vi "SwissSPAD Live_Decode SS2 FPGA Data_DVI.vi"(7 "SwissSPAD Live Gate Image Data Q":refnum<queue>, 8 "Error In":errorcluster, 9 "Buffer Size (#8-bit Images)":i32, 10 "SwissSPAD Live Internal Variables":T1={"okCFrontPanelDevices Refnum"=refnum, "Bottom Device Refnum"=refnum, "Display Image"=refnum, "# Live Images"=0, "relative s"=0.0, "# Image Sets"=0, "Message"="", "Current Image Set"=0, "# Datasets in Series"=0, "Current Dataset"=0, "Live Mode"=FALSE, "Recording Mode"=FALSE, "Record Button"=refnum, "\nLive Button"=refnum, "SwissSPAD Live Gate Image Data Q Name"="SS2 Live Gate Data Q", "Discard First Image"=FALSE, "Image Information"={"Save ROI Only"=FALSE, "Left"=0, "Top"=0, "Right"=0, "Bottom"=0, "Use Current ROI"=FALSE}, "Image Binning Options"={"Use Image Binning"=FALSE, "X Bin"=1, "Y Bin"=1}, "Bottom FPGA Serial Number"="", "Detector PCB Version"=enum."SS2 PCB1", "# Acquisitions"=1, "10 bits"=FALSE, "Top FPGA Serial Number"="", "Top Device Refnum"=refnum, "okCFrontPanel Refnum"=refnum} {"# Acquisitions" min=1; "Image Binning Options"."Y Bin" min=1; "Image Binning Options"."X Bin" min=1}, 11 "FPGA Data Q":refnum<queue>) -> ()   [LabVIEW 2021]
uses:
  SwissSPAD Live_Internal Variables.ctl
  D:/UCLA Thinkpad Google Drive/LabVIEW 2021 SP1/builds/SwissSPAD Live Distribution/Opal Kelly/C# Wrapper/v5.0.2/libFrontPanel-csharp.dll
  Opal Kelly/C# Wrapper/v5.0.2/libFrontPanel-csharp.dll
  <vilib>/vision/Image Controls.llb/IMAQ Image.ctl
  SwissSPAD Live_Image ROI Information.ctl
  Phasor/Image Binning Options.ctl
  SwissSPAD Live_SSx PCB Version.ctl
  8d2e2152-5180-46c7-ad9e-0233ef769053.vi
  LV Tools/Logical Processors Used.vi
  <vilib>/vision/NI_Vision_Development_Module.lvlib
  Notebook/Notebook.lvlib
  Rich Text Box/Rich Text Box.lvlib
panel:
  out "Activate Trigger Error Out":errorcluster
  out "8-bit Image Count":i32
  out "Error Out":errorcluster
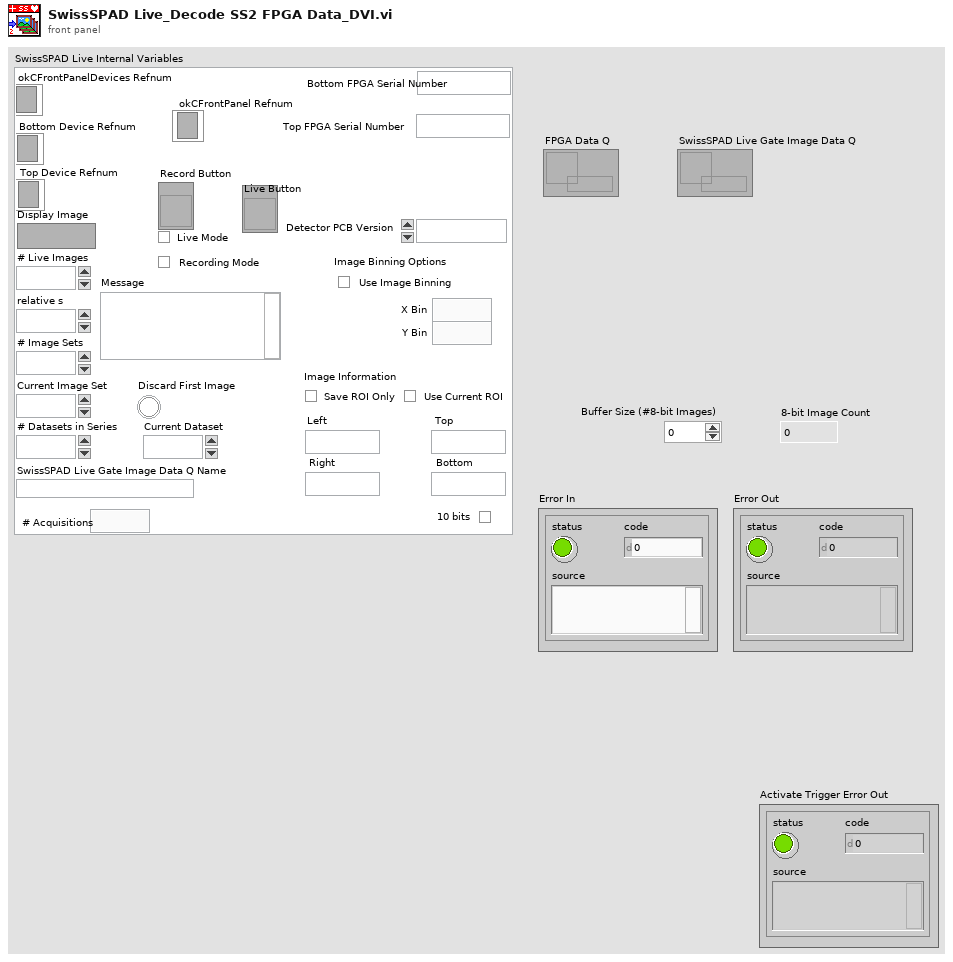
[diagram p1: front panel]
types:
  T1 = typedef "SwissSPAD Live_Internal Variables.ctl" = cluster{"okCFrontPanelDevices Refnum":refnum<k24>, "Bottom Device Refnum":refnum<k24>, "Display Image":T2, "# Live Images":i32, "relative s":dbl, "# Image Sets":i32, "Message":string, "Current Image Set":i32, "# Datasets in Series":i32, "Current Dataset":i32, "Live Mode":bool, "Recording Mode":bool, "Record Button":refnum<vi>, "\nLive Button":refnum<vi>, "SwissSPAD Live Gate Image Data Q Name":string, "Discard First Image":bool, "Image Information":T3, "Image Binning Options":T4, "Bottom FPGA Serial Number":string, "Detector PCB Version":T5, "# Acquisitions":u32, "10 bits":bool, "Top FPGA Serial Number":string, "Top Device Refnum":refnum<k24>, "okCFrontPanel Refnum":refnum<k24>}
  T2 = typedef "IMAQ Image.ctl" = refnum<image>
  T3 = typedef "SwissSPAD Live_Image ROI Information.ctl" = cluster{"Save ROI Only":bool, "Left":u16, "Top":u16, "Right":u16, "Bottom":u16, "Use Current ROI":bool}
  T4 = typedef "Image Binning Options.ctl" = cluster{"Use Image Binning":bool, "X Bin":i32, "Y Bin":i32}
  T5 = typedef "SwissSPAD Live_SSx PCB Version.ctl" = enum16{"unknown", "SS2 PCB1", "SS2 PCB2", "SS3 PCB1"}
  T6 = typedef "Image Type" = u32
  T7 = typedef "Rich Text Box.lvlib/Text Formatting.ctl" = cluster{"Font":string, "Text Color":T8, "Text Background Color":T8, "Text Style":enum16{"Regular", "Bold", "Italic", "Underline", "Strikeout"}, "Font Size (Points)":dbl, "Text Alignment":i32}
  T8 = typedef "Rich Text Box.lvlib/Text Colors.ctl" = enum16{"Unchanged", "Black", "Blue", "Brown", "Gray", "Green", "Orange", "Pink", "Red", "White"}
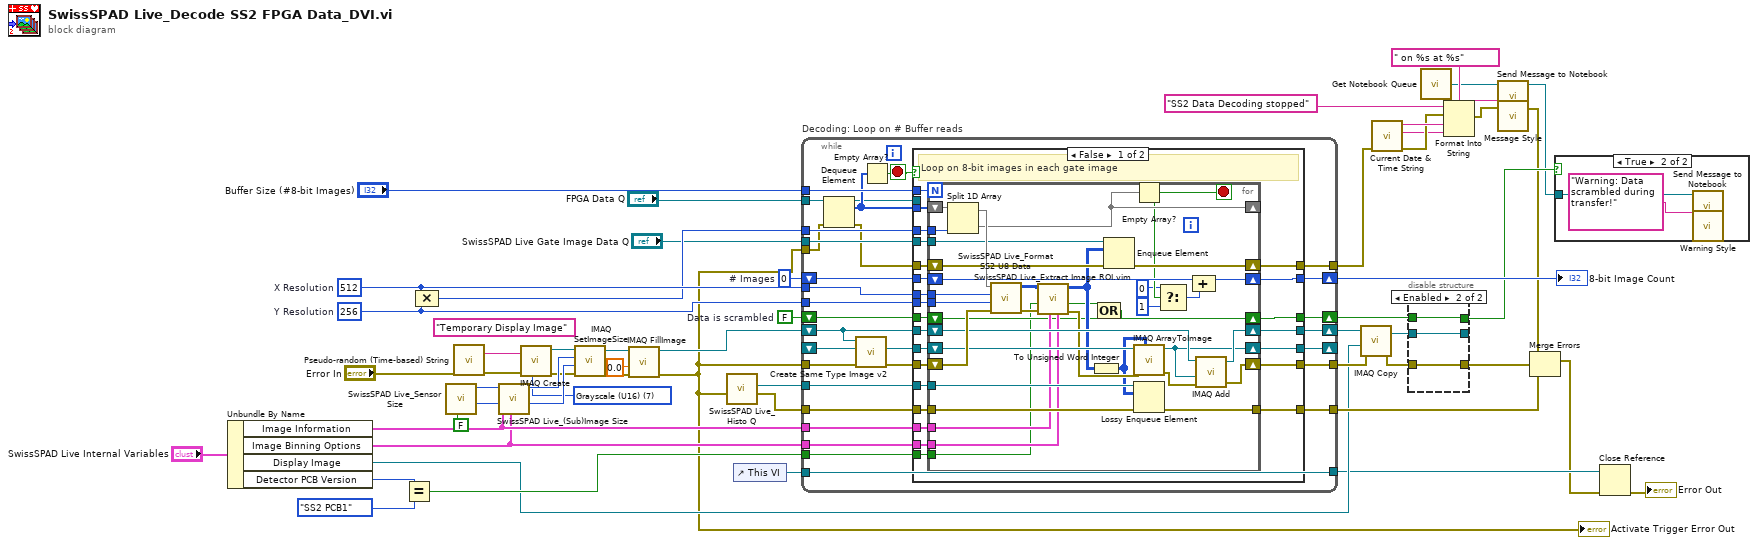
[diagram p0: block diagram]
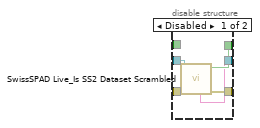
[diagram p2: hidden frame]
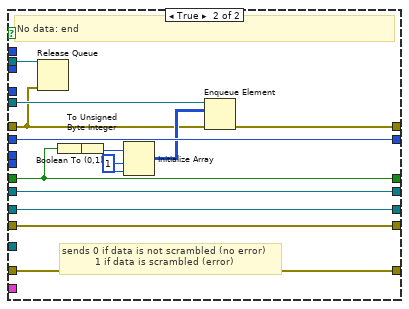
[diagram p4: hidden frame]
diagram:
  w32 = FALSE  # Data is scrambled
  w40 = T6 7 items=["Grayscale (U8)", "Grayscale (I16)", "Grayscale (SGL)", "Complex (CSG)", "RGB (U32)", "HSL (U32)", "RGB (U64)", "Grayscale (U16)"] ("Image Type")
  (unwired) "Temporary Display Image" ("Image Name")
  w54 = 0  # # Images
  w33 = 256  # Y Resolution
  w58 = 512  # X Resolution
  n1 = Unbundle By Name("SwissSPAD Live Internal Variables") -> ("Image Information"=w31:T3, "Image Binning Options"=w30:T4, "Display Image"=w24:T2, "Detector PCB Version"=w29:T5)
  n2 = Equal?(x=w29, y=SwissSPAD_Live_SSx_PCB_Version."SS2 PCB1" ("PCB Version")) -> (x = y?=w27:bool)
  n3 = Compound Arithmetic op=MULTIPLY(w58, w33) -> (w38:i32)
  n4 = call "SwissSPAD Live_Sensor Size.vi"("Set/Get(F)"=FALSE) -> ("Y size"=w41:i32, "X size"=w42:i32)  [unwired: 8 in, 1 out]
  n5 = call "Pseudo-random (Time-based) String.vi"("Error In"="Error In") -> ("Error Out"=w9:errorcluster, "result string"=w8:string)  [unwired: 9 in]
  n6 = call "SwissSPAD Live_(Sub)Image Size.vi"("Image Binning Options"=w30, "Image Information"=w31, "# Pixel Y in"=w41, "# Pixel X in"=w42) -> ("# Pixel Y out"=w52:i32, "# Pixel X out"=w53:i32)  [unwired: 6 in]
  n7 = call "IMAQ Create"("Image Name"=w8, "Image Type"=w40, "error in (no error)"=w9) -> ("New Image"=w49:T2, "error out"=w50:errorcluster)  [unwired: 2 in]
  n8 = call "IMAQ SetImageSize"("error in (no error)"=w50, "Y Resolution"=w52, "X Resolution"=w53, "Image"=w49) -> ("error out"=w47:errorcluster, "Image Out"=w48:T2)  [unwired: 1 in]
  n9 = call "IMAQ FillImage"("error in (no error)"=w47, "Pixel Value (U8, U16, I16, Float)"=sgl 0.0, "Image"=w48) -> ("error out"=w3:errorcluster, "Image Out"=w46:T2)  [unwired: 7 in]
  "Activate Trigger Error Out" <- w3
  n10 = call "SwissSPAD Live_Histo Q.vi"("error in (no error)"=w3) -> ("error out"=w56:errorcluster, "SS2 Live Histo Q"=w57:refnum<queue>)  [unwired: 5 in]
  n11 = control-ref of="This VI"() -> (w7:refnum<vi>)
  n12 = while "Decoding: Loop on # Buffer reads" {
    tunnel: w33 -> [w89]
    tunnel: w58 -> [w88]
    tunnel: w3 -> [w81]
    tunnel: "Buffer Size (#8-bit Images)" -> [w87]
    tunnel: w38 -> [w86]
    shift-right: [w72] -> _
    shift-left: _ -> [w84]
    tunnel: [w85] -> w43
    tunnel: "SwissSPAD Live Gate Image Data Q" -> [w79]
    tunnel: w3 -> [w70]
    tunnel: [w78] -> w16
    tunnel: w57 -> [w77]
    tunnel: w56 -> [w76]
    tunnel: [w75] -> w55
    shift-right: [w74] -> w44
    shift-left: w46 -> [w83]
    tunnel: "FPGA Data Q" -> [w71]
    shift-right: [w80] -> w51
    shift-left: w54 -> [w66]
    tunnel: w31 -> [w65]
    tunnel: w30 -> [w64]
    shift-right: [w63] -> w34
    shift-left: w32 -> [w62]
    tunnel: w27 -> [w61]
    tunnel: w7 -> [w59]
    tunnel: [w59] -> w6
    stop <- w67 stop-if-true
    n13 = Dequeue Element(queue=w71, error in (no error)=w70) -> (queue out=w60:refnum<queue>, element=w68:u8[], error out=w69:errorcluster)  [unwired: 1 in, 1 out]
    n14 = call "Create Same Type Image v2.vi"("error in (no error)"=w81, "Image Dst"=w84, "Image Src"=w83) -> ("error out"=w82:errorcluster, "Image Dst"=w73:T2)  [unwired: 6 in, 1 out]
    n15 = Empty Array?(array=w68) -> (empty?=w67:bool)
    n16 = case shown="False" w67 {
      tunnel: w89 -> [w113 _]
      tunnel: w88 -> [w112 _]
      tunnel: w87 -> [w111 _]
      tunnel: w86 -> [w110 _]
      tunnel: [w109 w160] -> w85
      tunnel: w83 -> [w108 w162]
      tunnel: w82 -> [w107 w160]
      tunnel: [w94 w163] -> w80
      tunnel: w79 -> [w106 w158]
      tunnel: [w105 w157] -> w78
      tunnel: w77 -> [w104 _]
      tunnel: w76 -> [w103 w159]
      tunnel: [w102 w159] -> w75
      tunnel: [w101 w162] -> w74
      tunnel: w73 -> [w100 w161]
      tunnel: [w99 w161] -> w72
      tunnel: w69 -> [w98 w150]
      tunnel: w68 -> [w97 _]
      tunnel: w66 -> [w95 w163]
      tunnel: w65 -> [w96 _]
      tunnel: w64 -> [w93 _]
      tunnel: [w91 w156] -> w63
      tunnel: w62 -> [w92 w156]
      tunnel: w61 -> [w90 _]
      tunnel: w60 -> [_ w151]
      frame False {
        # "Loop on 8-bit images in each gate image"
        n17 = for {
          N: w111 -> [_]
          tunnel: w113 -> [w149]
          tunnel: w112 -> [w148]
          shift-right: [w140] -> w109
          shift-left: w107 -> [w147]
          shift-right: [w139] -> _
          shift-left: w97 -> [w146]
          tunnel: w110 -> [w144]
          tunnel: w106 -> [w138]
          shift-right: [w136] -> w105
          shift-left: w98 -> [w137]
          tunnel: w104 -> [w135]
          tunnel: w103 -> [w134]
          tunnel: [w133] -> w102
          shift-right: [w132] -> w101
          shift-left: w108 -> [w142]
          shift-right: [w131] -> w99
          shift-left: w100 -> [w143]
          tunnel: w96 -> [w120]
          shift-right: [w125] -> w94
          shift-left: w95 -> [w126]
          tunnel: w93 -> [w119]
          shift-right: [w116] -> w91
          shift-left: w92 -> [w117]
          tunnel: w90 -> [w115]
          stop <- w124 stop-if-true
          n18 = Split 1D Array(array=w146, index=w144) -> (first subarray=w145:u8[], second subarray=w139:u8[])
          n19 = call "SwissSPAD Live_Format SS2 U8 Data.vi"("Error In"=w147, "Y Resolution"=w149, "X Resolution"=w148, "Flattened Image"=w145) -> ("Error Out"=w129:errorcluster, "Image out"=w130:u8[][])  [unwired: 6 in]
          n20 = call "SwissSPAD Live_Extract Image ROI.vim"("Image Binning Options"=w119, "Image Information"=w120, "Error In"=w129, "Test for scrambling"=w115, "Image in"=w130) -> ("Error Out"=w128:errorcluster, "Data is scrambled"=w118:bool, "Image out"=w127:u8[][])  [unwired: 4 in]
          n21 = To Unsigned Word Integer(number=w127) -> (unsigned 16bit integer=w114:u16[][])
          n22 = Compound Arithmetic op=OR(w118, w117) -> (w116:bool)
          n23 = Enqueue Element(queue=w138, element=w127, error in (no error)=w137) -> (error out=w136:errorcluster)  [unwired: 1 in, 2 out]
          n24 = Empty Array?(array=w139) -> (empty?=w124:bool)
          n25 = call "IMAQ ArrayToImage"("Image Pixels (U16)"=w114, "error in (no error)"=w128, "Image"=w143) -> ("error out"=w141:errorcluster, "Image Out"=w131:T2)  [unwired: 7 in]
          n26 = Lossy Enqueue Element(queue=w135, element=w114, error in (no error)=w134) -> (error out=w133:errorcluster)  [unwired: 3 out]
          n27 = Select(t=0 ("value"), s=w124, f=1) -> (s? t:f=w123:i32)
          n28 = Compound Arithmetic op=ADD(w126, w123) -> (w125:i32)
          n29 = call "IMAQ Add"("Image Src A"=w142, "Image Src B"=w131, "error in (no error)"=w141) -> ("Image Dst Out"=w132:T2, "error out"=w140:errorcluster)  [unwired: 4 in]
        }
      }
      frame True {
        w153 = 1 ("dimension size")
        # "sends 0 if data is not scrambled (no error)\n           1 if data is scrambled (error)"
        # "No data: end"
        n30 = Release Queue(queue=w151, error in (no error)=w150) -> ()  [unwired: 1 in, 3 out]
        n31 = Boolean To (0,1)(Boolean=w156) -> (0, 1=w155:i16)
        n32 = To Unsigned Byte Integer(number=w155) -> (unsigned 8bit integer=w154:u8)
        n33 = Initialize Array(w154, w153, w153) -> (w152:u8[][])
        n34 = Enqueue Element(queue=w158, element=w152, error in (no error)=w150) -> (error out=w157:errorcluster)  [unwired: 1 in, 2 out]
      }
    }
  }
  "8-bit Image Count" <- w51
  n35 = call "IMAQ Copy"("error in (no error)"=w43, "Image Dst"=w24, "Image Src"=w44) -> ("error out"=w37:errorcluster, "Image Dst Out"=w25:T2)  [unwired: 3 in]
  n36 = call "Current Date & Time String.vi"("Error In"=w16) -> ("Error Out"=w15:errorcluster, "time string"=w12:string, "date string"=w20:string)  [unwired: 8 in]
  n37 = disable-structure shown="Enabled" {
    disable-tunnel: w37 -> [w168 w170]
    disable-tunnel: [w167 w170] -> w36
    disable-tunnel: w25 -> [w166 w171]
    disable-tunnel: [w165 w169] -> w35
    disable-tunnel: [w164 w171] -> _
    disable-tunnel: w34 -> [_ w169]
    frame Disabled {
      n38 = call "SwissSPAD Live_Is SS2 Dataset Scrambled.vi"("Error In"=w168, "Refnum in"=w166) -> ("Error Out"=w167:errorcluster, "SS2 image is scrambled"=w165:bool, "Warning"=w164:string)  [unwired: 4 in, 3 out]
    }
    frame Enabled {
    }
  }
  n39 = call "Get Notebook Queue.vi"() -> ("Notebook Queue"=w17:refnum<queue>)  [unwired: 9 in]
  n40 = Format Into String(format string=" on %s at %s", initial string="SS2 Data Decoding stopped" ("Message"), error in=w15, w20, w12) -> (resulting string=w19:string, error out=w14:errorcluster)
  n41 = call "Message Style.vi"() -> ("Message Formatting"=w18:T7)
  n42 = call "Send Message to Notebook.vi"("Text Formatting"=w18, "Error In"=w14, "Message"=w19, "Notebook Queue"=w17) -> ("Error Out"=w13:errorcluster, "Notebook Queue"=w1:refnum<queue>)  [unwired: 4 in]
  n43 = Merge Errors(w13, w36, w55) -> (w5:errorcluster)
  n44 = case shown="True" w35 {
    tunnel: w1 -> [_ w172]
    frame False {
    }
    frame True {
      n45 = call "Warning Style.vi"() -> ("Error Formatting"=w174:T7)
      n46 = call "Send Message to Notebook.vi"("Text Formatting"=w174, "Message"="Warning: Data scrambled during transfer!" ("format string"), "Notebook Queue"=w172) -> ()  [unwired: 5 in, 2 out]
    }
  }
  n47 = Close Reference(reference=w6, error in (no error)=w5) -> (error out=→"Error Out":errorcluster)
